vi "Non Linear Fit.vi"(10 "X":dbl[](array[numeric]), 11 "Y":dbl[](array[numeric])) -> (2 "Non Linear Model":dbl[](array[numeric]), 3 "Fit Verification":cluster{dbl[], "Best Power Fit":dbl[]}[](array[cluster]))   [LabVIEW 2013, in "AvaSpec.lvlib" / "AvaSpec Logging.lvlib"]
uses:
  AvaSpec Logging.lvlib
  <vilib>/gmath/NumericalOptimization/Nonlinear Curve Fit LM formula string.vi
  <vilib>/gmath/NI_Gmath.lvlib
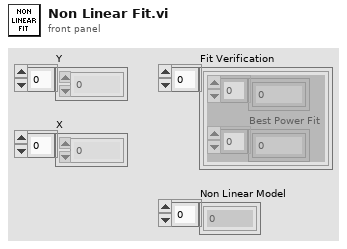
[diagram p1: front panel]
types:
  T1 = cluster{"model":string, "Parameters":string[], "x":string}
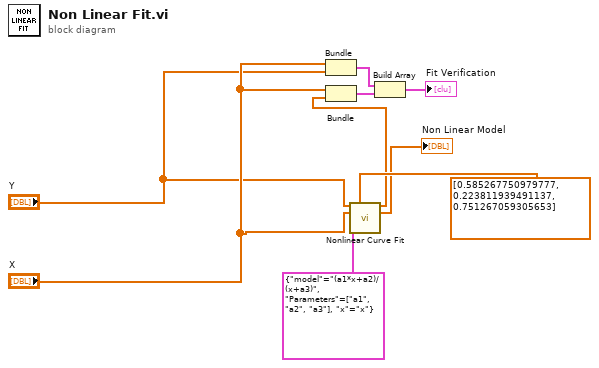
[diagram p0: block diagram]
diagram:
  n1 = Bundle("X"="X", "Y"="Y") -> (w7:cluster{"X":dbl[], "Y":dbl[]})  [unwired: 1 in]
  n2 = call-poly <vilib>:"Nonlinear Curve Fit.vi"("Y"="Y", "initial parameters"=dbl[] [0.585267750979777, 0.223811939491137, 0.751267059305653], "X"="X", "model description"=T1 {"model"="(a1*x+a2)/(x+a3)", "Parameters"=["a1", "a2", "a3"], "x"="x"}) -> ("best nonlinear fit"=w2:dbl[], "best fit parameters"=→"Non Linear Model":dbl[])  [unwired: 7 in, 3 out]
  n3 = Bundle("X"="X", "best nonlinear fit"=w2) -> (w8:cluster{"X":dbl[], "best nonlinear fit":dbl[]})  [unwired: 1 in]
  n4 = Build Array(w7, w8) -> (→"Fit Verification":cluster{"X":dbl[], "best nonlinear fit":dbl[]}[])
